vi "Set Or Reset Bit(U32).vi"(8 "error in (no error)":errorcluster caption="错误输入（无错误）", 10 "Bit(0-31)":i32, 11 "Input(U32)":u32 format="%.0x") -> (0 "error out":errorcluster caption="错误输出", 3 "Output(32)":u32 format="%.0x")   [LabVIEW 2012]
panel:
  in  "Set and Reset":bool
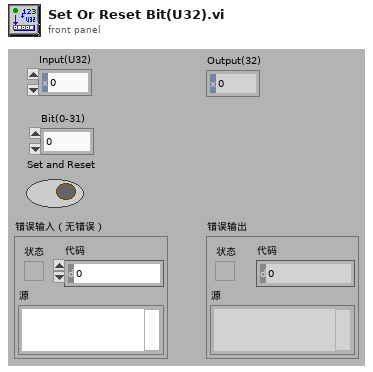
[diagram p1: front panel]
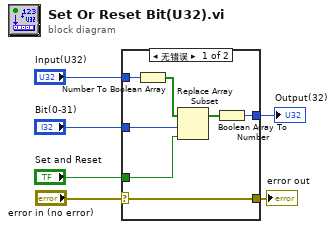
[diagram p0: block diagram]
diagram:
  n1 = case shown="无错误" "error in (no error)" {
    selector: "error in (no error)" -> [w13 w14]
    tunnel: [w13 w14] -> w5
    tunnel: "Bit(0-31)" -> [w9 _]
    tunnel: "Input(U32)" -> [w12 _]
    tunnel: "Set and Reset" -> [w10 _]
    tunnel: [w7 _] -> w1
    frame No Error {
      n2 = Number To Boolean Array(number=w12) -> (Boolean array=w11:bool[])
      n3 = Replace Array Subset(array=w11, new element=w10, index=w9) -> (w8:bool[])
      n4 = Boolean Array To Number ("布尔数组至数值转换")(Boolean array=w8) -> (number=w7:u32)
    }
    frame Error {
    }
  }
  "error out" <- w5
  "Output(32)" <- w1
